vi "ComputeBeadValidity.vi"(10 "Image Pixels (U8)":u8[][](array[numeric])) -> (3 "Bead validity":dbl)   [LabVIEW 2011]
uses:
  <vilib>/Analysis/NI_AALBase.lvlib
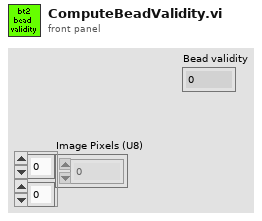
[diagram p1: front panel]
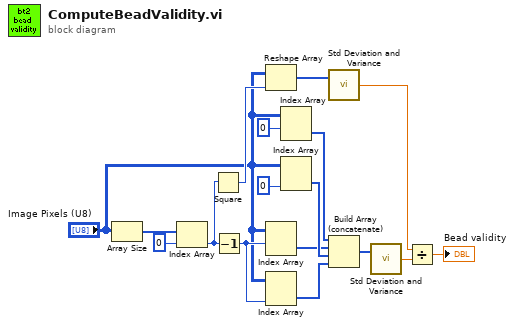
[diagram p0: block diagram]
diagram:
  n1 = Array Size(array="Image Pixels (U8)") -> (size(s)=w3:i32[])
  n2 = Index Array(array=w3, index=0) -> (element=w1:i32)
  n3 = Square(x=w1) -> (x^2=w16:i32)
  n4 = Decrement(x=w1) -> (x-1=w10:i32)
  n5 = Reshape Array("Image Pixels (U8)", w16) -> (w17:u8[])
  n6 = Index Array(array="Image Pixels (U8)", index (row)=w10) -> (element=w12:u8[])  [unwired: 1 in]
  n7 = Index Array(array="Image Pixels (U8)", index (col)=w10) -> (element=w14:u8[])  [unwired: 1 in]
  n8 = Index Array(array="Image Pixels (U8)", index (row)=0) -> (element=w11:u8[])  [unwired: 1 in]
  n9 = Index Array(array="Image Pixels (U8)", index (col)=0 ("disabled index (col)")) -> (element=w13:u8[])  [unwired: 1 in]
  n10 = call <vilib>:"Std Deviation and Variance.vi"("X"=w17) -> ("standard deviation"=w6:dbl)  [unwired: 1 in, 2 out]
  n11 = Build Array (concatenate)(w11, w12, w13, w14) -> (w15:u8[])
  n12 = call <vilib>:"Std Deviation and Variance.vi"("X"=w15) -> ("standard deviation"=w7:dbl)  [unwired: 1 in, 2 out]
  n13 = Divide(x=w6, y=w7) -> (x/y=→"Bead validity":dbl)
